vi "resultsDuplicateChs.vi"(5 "Give non duplicate inst values each row?":bool, 7 "dupsArray":i32[](array[numeric]), 8 "Number of Initial Channels":i32, 10 "chValuesIn":string[](array[string]), 11 "chNamesIn":string[](array[string])) -> (1 "rowSplitting":string[][](array[string]), 2 "chValuesOut":string[](array[string]), 3 "chNamesOut":string[](array[string]), 4 "valsToKeepinDups":bool[](array[boolean]))   [LabVIEW 2020]
uses:
  Globals/Meas_global.vi
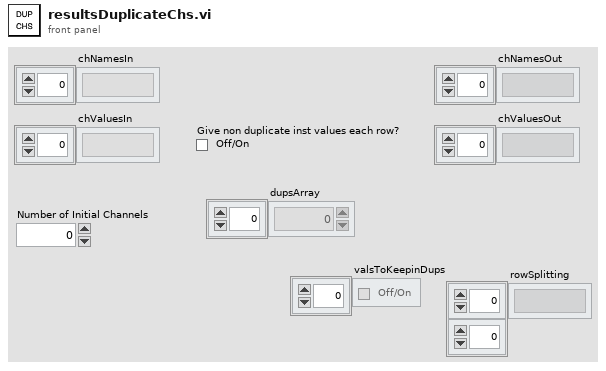
[diagram p1: front panel]
types:
  T1 = typedef "Analysis_info_cluster.ctl" = cluster{"Colour":u32, "Inst type":T2, "Inst name":string, "Symbol":string, "Code name":string, "Extra Info":string, "Inst Array":T3, "Extra Titles":string[], "Extra Values":string[], "U":dbl, "u^2":dbl, "u^3":dbl, "u^4":dbl, "Skew_u":dbl, "Kurt_u":dbl, "Sd Error in Mean":dbl, "% u'/U":dbl, "X":dbl, "Y":dbl, "Z":dbl, "Timescale integral Estimate":dbl, "Sd Error in Variance":dbl, "Calib File":path, "Calib Constants":dbl[], "Output Position":bool, "Stats":enum16{"None", "Basic", "Full"}, "Av Sampling Rate":dbl, "Av No of Samples":dbl, "Total Meas Time (s)":dbl, "ADAM Ch Name":string, "Max value":dbl, "Min value":dbl, "Req Sample Rate Hz":dbl, "Sync Delay Time (s)":dbl, "Ch No":i16, "Device":string, "Use Latest Calib":bool, "Port":string, "Metadata Ch Names":string[], "Metadata Ch Values":string[], "Label":string}
  T2 = typedef "Inst_type.ctl" = enum16{"Raw voltage", "Raw with zero offsetting", "Propeller anemometer", "Pressure Transducer", "Pitot-static tube", "Hot wire", "Cross wire 1", "Cross wire 2", "Generic Linear", "Generic Polynomial", "Generic BackPoly", "Fast FID", "Thermocouple", "Cold wire", "Pulsed Wire", "LDA Vel", "LDA Tran time", "LDA Arr time", "Microphone"}
  T3 = typedef "Instrument_Array.ctl" = enum16{"PWA", "LDA", "Analogue"}
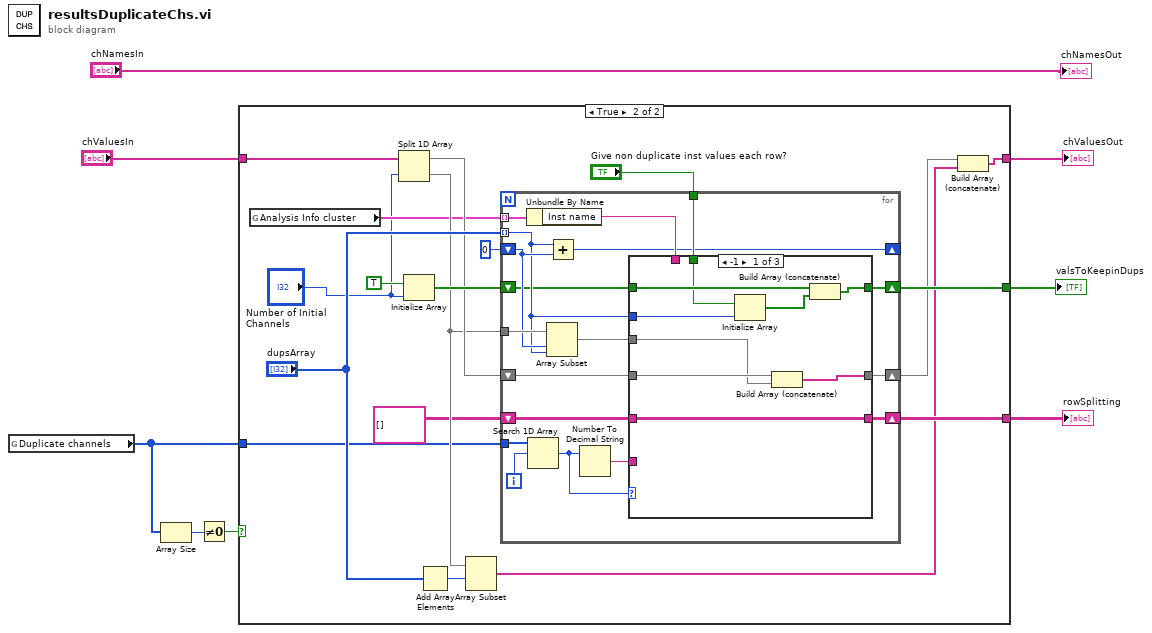
[diagram p0: block diagram]
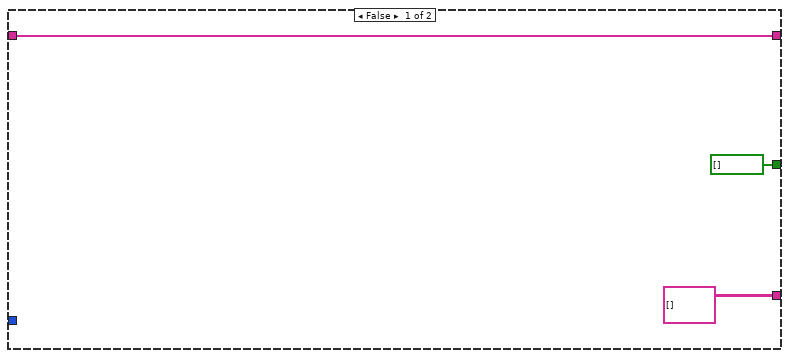
[diagram p2: hidden frame]
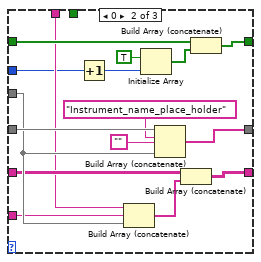
[diagram p3: hidden frame]
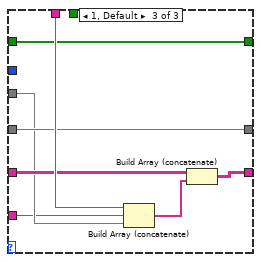
[diagram p4: hidden frame]
diagram:
  n1 = global read "Meas_global.vi" "Duplicate channels"() -> (w3:i32[])
  n2 = Array Size(array=w3) -> (size(s)=w4:i32)
  n3 = Not Equal To 0?(x=w4) -> (x != 0?=w2:bool)
  n4 = case shown="True" w2 {
    tunnel: [w11 w29] -> w8
    tunnel: [string[][] [] w28] -> w7
    tunnel: [bool[] [] w26] -> w6
    tunnel: "chValuesIn" -> [w11 w21]
    tunnel: w3 -> [_ w13]
    frame False {
    }
    frame True {
      n5 = global read "Meas_global.vi" "Analysis Info cluster"() -> (w14:T1[])
      n6 = Split 1D Array(array=w21, index="Number of Initial Channels") -> (first subarray=w18:string[], second subarray=w16:string[])
      n7 = Initialize Array(TRUE, "Number of Initial Channels") -> (w25:bool[])
      n8 = Add Array Elements(numeric array="dupsArray") -> (sum=w17:i32)
      n9 = Array Subset(array=w16, index=w17) -> (w23:string[])  [unwired: 1 in]
      n10 = for {
        shift-right: [w45] -> w22
        shift-left: w18 -> [w46]
        tunnel: "dupsArray" -> [w37] mode=indexing
        tunnel: w16 -> [w47]
        shift-right: [w33] -> _
        shift-left: 0 -> [w44]
        tunnel: w13 -> [w42]
        shift-right: [w41] -> w28
        shift-left: string[][] [] -> [w40]
        tunnel: w14 -> [w38] mode=indexing
        shift-right: [w35] -> w26
        shift-left: w25 -> [w36]
        tunnel: "Give non duplicate inst values each row?" -> [w34]
        i -> [w32]
        n11 = Unbundle By Name(w38) -> ("Inst name"=w39:string)
        n12 = Search 1D Array(1D array=w42, element=w32) -> (index of element=w30:i32)  [unwired: 1 out]
        n13 = Array Subset(array=w47, index=w44, length=w37) -> (w43:string[])
        n14 = Add(x=w37, y=w44) -> (x+y=w33:i32)
        n15 = Number To Decimal String(number=w30) -> (decimal integer string=w31:string)  [unwired: 1 in]
        n16 = case shown="-1" w30 {
          tunnel: w46 -> [w56 w71 w76]
          tunnel: [w55 w72 w76] -> w45
          tunnel: w43 -> [w54 w70 w74]
          tunnel: w39 -> [_ w62 w80]
          tunnel: [w53 w68 w78] -> w41
          tunnel: w40 -> [w53 w67 w77]
          tunnel: w37 -> [w52 w60 _]
          tunnel: w36 -> [w50 w65 w75]
          tunnel: [w49 w64 w75] -> w35
          tunnel: w34 -> [w48 _ _]
          tunnel: w31 -> [_ w61 w73]
          frame -1 {
            n17 = Initialize Array(w48, w52) -> (w51:bool[])
            n18 = Build Array (concatenate)(w56, w54) -> (w55:string[])
            n19 = Build Array (concatenate)(w50, w51) -> (w49:bool[])
          }
          frame 0 {
            n20 = Increment(x=w60) -> (x+1=w59:i32)
            n21 = Build Array (concatenate)(w62, w61, w70) -> (w69:string[])
            n22 = Initialize Array(TRUE, w59) -> (w63:bool[])
            n23 = Build Array (concatenate)(w71, "Instrument_name_place_holder", "", w70) -> (w72:string[])
            n24 = Build Array (concatenate)(w67, w69) -> (w68:string[][])
            n25 = Build Array (concatenate)(w65, w63) -> (w64:bool[])
          }
          frame 1, Default {
            n26 = Build Array (concatenate)(w80, w73, w74) -> (w79:string[])
            n27 = Build Array (concatenate)(w77, w79) -> (w78:string[][])
          }
        }
      }
      n28 = Build Array (concatenate)(w22, w23) -> (w29:string[])
    }
  }
  "chValuesOut" <- w8
  "rowSplitting" <- w7
  "valsToKeepinDups" <- w6
  "chNamesOut" <- "chNamesIn"
